vi "Send End of Data Message.vi"   [LabVIEW 2013]
uses:
  Single Sector Pixel Cluster.ctl
  <vilib>/rvi/Emulation/niFpgaSctlEmulationGetInTimedLoop.vi
  <vilib>/rvi/DataTransferAndStorage/Container/Common/niFpgaContainerGetUniqueNameForEmu.vi
  <vilib>/rvi/FIFO/Fifo_Resource/nirvififoEmulationSetSize.vi
  <vilib>/rvi/errors/niFpgaSetErrorForExecOnDevCompSimple.vi
  <vilib>/rvi/eio/common/nirviEmuReportErrorAndStop.vi
  <vilib>/rvi/Emulation/niFpgaSctlEmulationFifoFullMgr.vi
  <vilib>/rvi/Emulation/niFpgaSctlEmulationResourceMgr.vi
  <vilib>/rvi/DataTransferAndStorage/Container/XNode/niFpgaContainer.xnode
  <vilib>/rvi/FIFO/Fifo_Resource/nirvififoEmulationWrite.vi
types:
  T1 = typedef "Single Sector Pixel Cluster.ctl" = cluster{"Sector #":u8, "Pixel Value":u8}
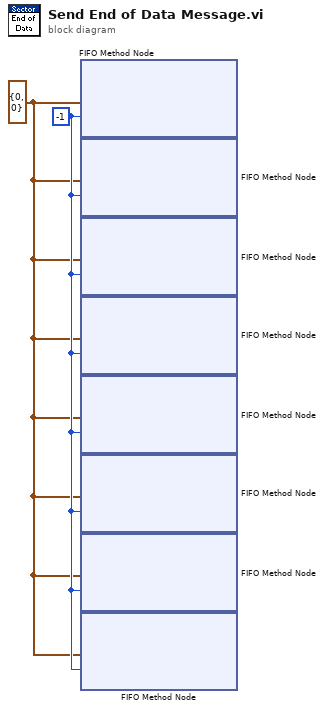
[diagram p0: block diagram]
diagram:
  w2 = -1 ("Timeout")
  w1 = T1 {"Sector #"=0, "Pixel Value"=0} ("Single Sector Pixel")
  n1 = xnode ("FIFO Method Node")("Element"=w1, "Timeout"=w2) -> ()  [unwired: 1 in, 2 out]
  n2 = xnode ("FIFO Method Node")("Element"=w1, "Timeout"=w2) -> ()  [unwired: 1 in, 2 out]
  n3 = xnode ("FIFO Method Node")("Element"=w1, "Timeout"=w2) -> ()  [unwired: 1 in, 2 out]
  n4 = xnode ("FIFO Method Node")("Element"=w1, "Timeout"=w2) -> ()  [unwired: 1 in, 2 out]
  n5 = xnode ("FIFO Method Node")("Element"=w1, "Timeout"=w2) -> ()  [unwired: 1 in, 2 out]
  n6 = xnode ("FIFO Method Node")("Element"=w1, "Timeout"=w2) -> ()  [unwired: 1 in, 2 out]
  n7 = xnode ("FIFO Method Node")("Element"=w1, "Timeout"=w2) -> ()  [unwired: 1 in, 2 out]
  n8 = xnode ("FIFO Method Node")("Element"=w1, "Timeout"=w2) -> ()  [unwired: 1 in, 2 out]
